vi "Read_Benchmark.vi"() -> ()   [LabVIEW 2017]
uses:
  <vilib>/NI_Real-Time Target Support.lvlib
  <resource>/objmgr/nimcai.rc
panel:
  out "Position Setpoint":dbl
  out "Mean time (us)":dbl format="%.3g"
  in  "Warmup iterations":i32=10
  in  "Calibrate?":bool
  out "Execution histogram":T1(graph)
  out "Standard deviation (us)":dbl format="%.3g"
  out "Max jitter (us)":dbl format="%.3g"
  out "Execution times (us)":dbl[](graph)
  in  "Iterations":i32=1000
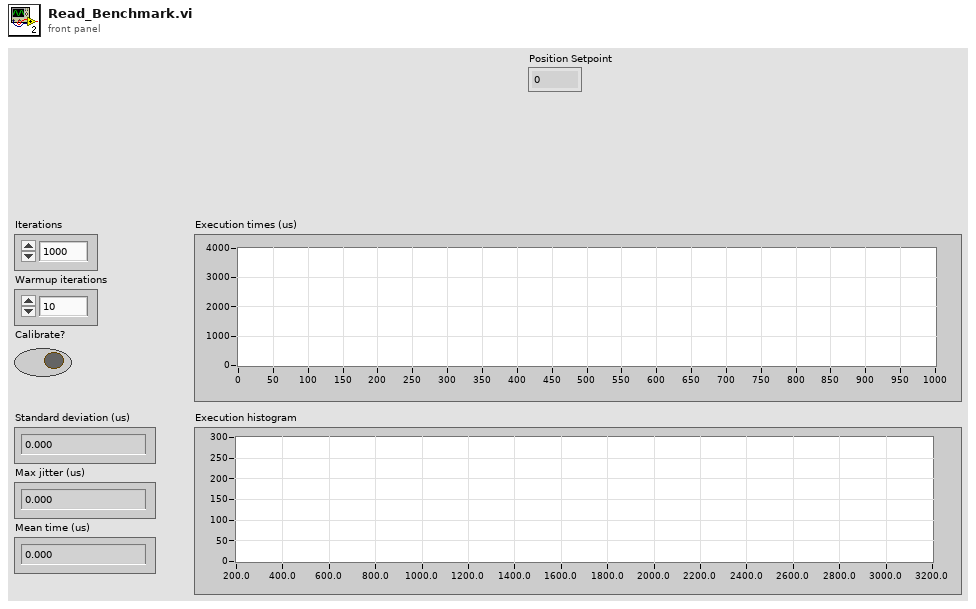
[diagram p1: front panel]
types:
  T1 = cluster{"X Values":dbl[], "Histogram: h(x)":i32[]}
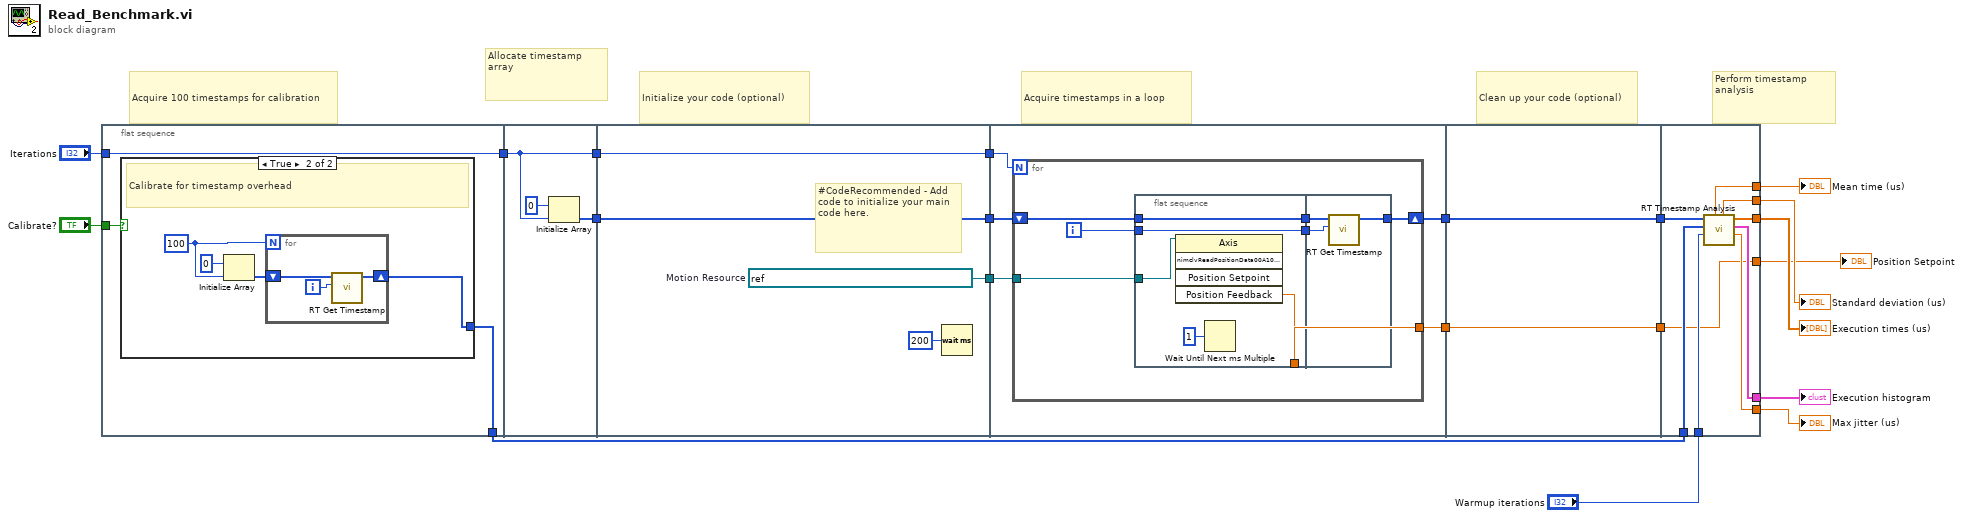
[diagram p0: block diagram]
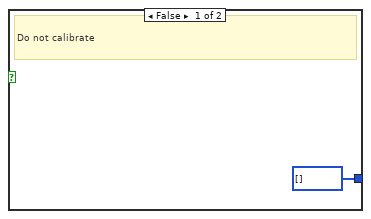
[diagram p2: hidden frame]
diagram:
  # "Perform timestamp analysis"
  # "Clean up your code (optional)"
  # "Acquire timestamps in a loop"
  # "Initialize your code (optional)"
  # "Allocate timestamp array"
  # "Acquire 100 timestamps for calibration"
  n1 = flat-sequence {
    tunnel: "Iterations" -> [w23]
    tunnel: [w23] -> w20
    tunnel: "Calibrate?" -> [w22]
    tunnel: [w21] -> w11
    tunnel: [w33] -> w19
    tunnel: [w34] -> w18
    tunnel: w20 -> [w33]
    tunnel: [w38] -> w17
    tunnel: [w37] -> w16
    tunnel: w19 -> [w38]
    tunnel: w18 -> [w37]
    tunnel: [w35] -> w4
    tunnel: [w43] -> w15
    tunnel: w17 -> [w42]
    tunnel: w16 -> [w41]
    tunnel: w4 -> [w40]
    tunnel: [w39] -> w3
    tunnel: w15 -> [w60]
    tunnel: [w60] -> w14
    tunnel: w3 -> [w59]
    tunnel: [w59] -> w1
    tunnel: w14 -> [w69]
    tunnel: w11 -> [w68]
    tunnel: [w67] -> w5
    tunnel: [w66] -> w9
    tunnel: [w65] -> w8
    tunnel: [w64] -> w10
    tunnel: "Warmup iterations" -> [w63]
    tunnel: [w62] -> w6
    tunnel: [w61] -> w2
    tunnel: w1 -> [w61]
    frame #0 {
      n2 = case shown="True" w22 {
        tunnel: [u64[] [] w28] -> w21
        frame False {
          # "Do not calibrate"
        }
        frame True {
          w26 = 100
          # "Calibrate for timestamp overhead"
          n3 = Initialize Array(u64 0, w26) -> (w27:u64[])
          n4 = for {
            N: w26 -> [_]
            shift-right: [w29] -> w28
            shift-left: w27 -> [w30]
            i -> [w31]
            n5 = call <vilib>:"RT Get Timestamp.vi"("iteration"=w31, "timestamp array in"=w30) -> ("timestamp array out"=w29:u64[])  [unwired: 1 in, 8 out]
          }
        }
      }
    }
    frame #1 {
      n6 = Initialize Array(u64 0, w33) -> (w34:u64[])
    }
    frame #2 {
      w35 = refnum<k21> "nism://RT CompactRIO Target/Axis 1"  # Motion Resource
      # "#CodeRecommended - Add code to initialize your main code here."
      n7 = Wait (ms)(milliseconds to wait=u32 200) -> ()  [unwired: 1 out]
    }
    frame #3 {
      n8 = for {
        N: w42 -> [_]
        shift-right: [w50] -> w43
        shift-left: w41 -> [w49]
        tunnel: w40 -> [w45]
        tunnel: [w44] -> w39
        i -> [w48]
        n9 = flat-sequence {
          tunnel: w49 -> [w55]
          tunnel: [w55] -> w47
          tunnel: w48 -> [w54]
          tunnel: [w54] -> w46
          tunnel: w45 -> [w53]
          tunnel: [w52] -> w44
          tunnel: [w58] -> w50
          tunnel: w47 -> [w56]
          tunnel: w46 -> [w57]
          frame #0 {
            n10 = invoke class="Axis" method="nimclvReadPositionData00A10001"(reference=w53) -> ("Position Feedback"=w52:dbl)  [unwired: 4 in, 4 out]
            n11 = Wait Until Next ms Multiple(millisecond multiple=u32 1) -> ()  [unwired: 1 out]
          }
          frame #1 {
            n12 = call <vilib>:"RT Get Timestamp.vi"("iteration"=w57, "timestamp array in"=w56) -> ("timestamp array out"=w58:u64[])  [unwired: 1 in, 8 out]
          }
        }
      }
    }
    frame #4 {
    }
    frame #5 {
      n13 = call <vilib>:"RT Timestamp Analysis.vi"("warmup iterations"=w63, "calibration array"=w68, "timestamp array"=w69) -> ("max jitter (uS)"=w66:dbl, "execution histogram"=w67:T1, "execution times (uS)"=w64:dbl[], "standard deviation (uS)"=w65:dbl, "mean time (uS)"=w62:dbl)  [unwired: 1 in, 3 out]
    }
  }
  "Execution times (us)" <- w10
  "Max jitter (us)" <- w9
  "Standard deviation (us)" <- w8
  "Execution histogram" <- w5
  "Mean time (us)" <- w6
  "Position Setpoint" <- w2
